vi "例6-9.vi"() -> ()   [LabVIEW 2019]
uses:
  <vilib>/Analysis/2dsp.llb/1D Auto Correlation (DBL).vi
  <vilib>/Analysis/NI_AALBase.lvlib
  <vilib>/Analysis/NI_AALPro.lvlib
panel:
  in  "噪声幅值":dbl=1.0
  in  "采样点数":dbl=1000.0
  in  "采样频率":dbl=1000.0
  in  "信号频率":dbl=10.0
  out "自相关图":cluster{dbl, i32, "Rxx":dbl[]}(graph)
  out "混合信号波形图":dbl[](graph)
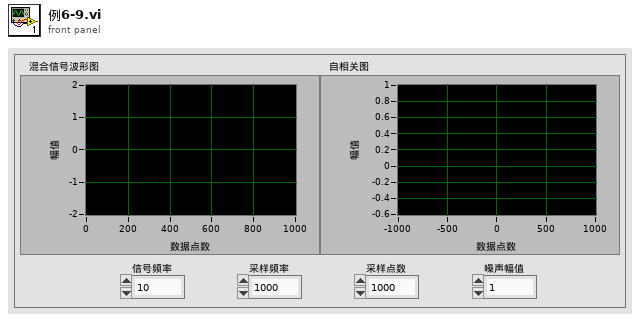
[diagram p1: front panel]
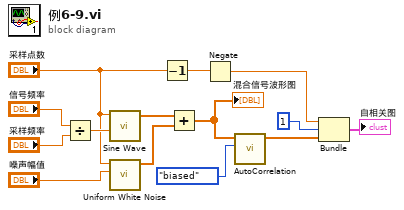
[diagram p0: block diagram]
diagram:
  n1 = Divide(x="信号频率", y="采样频率") -> (x/y=w12:dbl)
  n2 = call <vilib>:"Sine Wave.vi"("samples"="采样点数", "frequency"=w12) -> ("sine wave"=w11:dbl[])  [unwired: 3 in, 2 out]
  n3 = call <vilib>:"Uniform White Noise.vi"("amplitude"="噪声幅值", "samples"="采样点数") -> ("uniform white noise"=w10:dbl[])  [unwired: 8 in, 1 out]
  n4 = Decrement(x="采样点数") -> (x-1=w5:dbl)
  n5 = Add(x=w11, y=w10) -> (x+y=w9:dbl[])
  "混合信号波形图" <- w9
  n6 = Negate(x=w5) -> (-x=w4:dbl)
  n7 = call-poly <vilib>:"AutoCorrelation.vi"("normalization"=enum32{"none", "unbiased", "biased"}."biased", "X"=w9) -> ("Rxx"=w3:dbl[])  [unwired: 8 in, 1 out]
  n8 = Bundle(w4, 1, "Rxx"=w3) -> (→"自相关图":cluster{dbl, i32, "Rxx":dbl[]})  [unwired: 1 in]
